vi "Validate-Repair Path.vi"(11 "path in":string) -> (0 "Valid":bool, 1 "Path type":T1=enum."path-abempty", 2 "Segments":string[](array[string]), 3 "path out":string)   [LabVIEW 2013, in "openURI.lvlib" / "URI-Component.Path.lvclass"]
uses:
  URI-Component.Path.lvclass
  path type -- enum.ctl
  utilities/isHEXDigit.vi
  <vilib>/regexp/Match Regular Expression.xnode
  openURI.lvlib
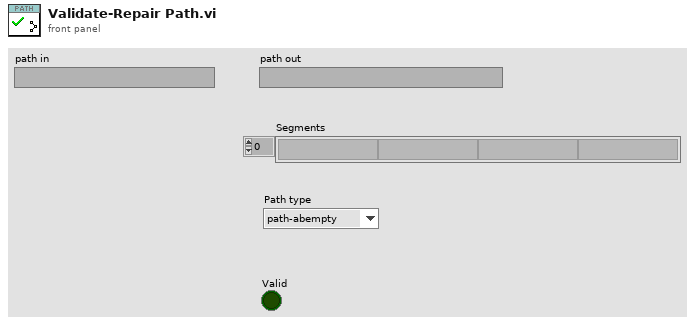
[diagram p1: front panel]
types:
  T1 = typedef "openURI.lvlib/URI-Component.Path.lvclass/path type -- enum.ctl" = enum16{"invalid", "path-abempty", "path-absolute", "path-noscheme", "path-rootless", "path-empty"}
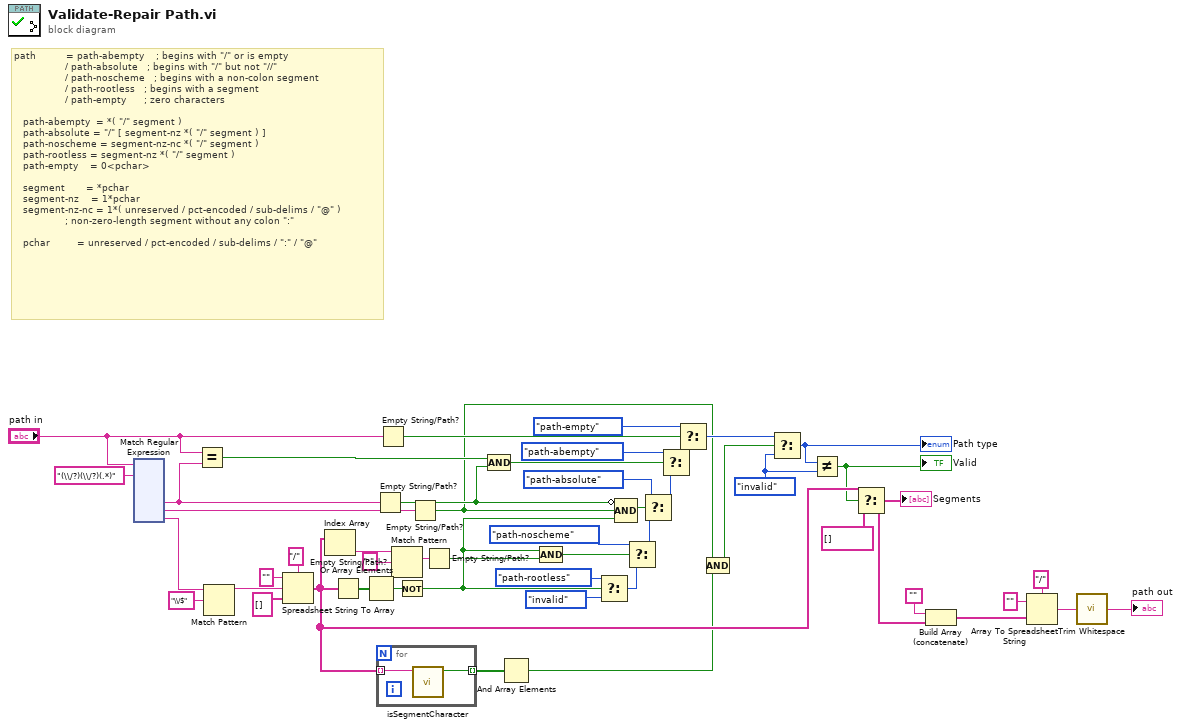
[diagram p0: block diagram]
diagram:
  w49 = path_type_--_enum."invalid" ("path type")
  # "path          = path-abempty    ; begins with \"/\" or is empty\n                 / path-absolute   ; begins with \"/\" but not \"//\"\n                 / path-noscheme   ; begins with a non-colon segment\n                 / path-rootless   ; begins with a segment\n                 / path-empty      ; zero characters\n\n   path-abempty  = *( \"/\" segment )\n   path-absolute = \"/\" [ segment-nz *( \"/\" segment ) ]\n   path-noscheme = segment-nz-nc *( \"/\" segment )\n   path-rootless = segment-nz *( \"/\" segment )\n   path-empty    = 0<pchar>\n\n   segment       = *pchar\n   segment-nz    = 1*pchar\n   segment-nz-nc = 1*( unreserved / pct-encoded / sub-delims / \"@\" )\n                 ; non-zero-length segment without any colon \":\"\n\n   pchar         = unreserved / pct-encoded / sub-delims / \":\" / \"@\""
  n1 = xnode "Match Regular Expression"("input string"="path in", "regular expression"="(\\/?)(\\/?)(.*)") -> ("submatch 1"=w19:string, "submatch 2"=w18:string, "submatch 3"=w40:string)  [unwired: 4 in, 5 out]
  n2 = Equal?(x="path in", y=w19) -> (x = y?=w22:bool)
  n3 = Match Pattern(string=w40, regular expression="\\/$") -> (before substring=w41:string)  [unwired: 1 in, 3 out]
  n4 = Spreadsheet String To Array(delimiter (Tab)="/", format string="", spreadsheet string=w41, array type (2D Dbl)=string[] [] ("Segments")) -> (array=w12:string[])
  n5 = Index Array(array=w12) -> (element=w47:string)  [unwired: 1 in]
  n6 = Empty String/Path?(string/path=w12) -> (empty?=w48:bool[])
  n7 = Or Array Elements(Boolean array=w48) -> (logical OR=w38:bool)
  n8 = Empty String/Path?(string/path=w19) -> (empty?=w34:bool)
  n9 = for {
    tunnel: [w52] -> w15 mode=indexing
    tunnel: w12 -> [w51] mode=indexing
    n10 = call "isSegmentCharacter.vi"("characters"=w51) -> ("pchar"=w52:bool)  [unwired: 10 in]
  }
  n11 = Empty String/Path?(string/path="path in") -> (empty?=w26:bool)
  n12 = Match Pattern(string=w47, regular expression=":" ("string")) -> (match substring=w43:string)  [unwired: 1 in, 3 out]
  n13 = Not(x=w38) -> (.not. x?=w45:bool)
  n14 = Empty String/Path?(string/path=w18) -> (empty?=w14:bool)
  n15 = Empty String/Path?(string/path=w43) -> (empty?=w44:bool)
  n16 = Compound Arithmetic op=AND(w22, w34) -> (w21:bool)
  n17 = And Array Elements(Boolean array=w15) -> (logical AND=w11:bool)
  n18 = Compound Arithmetic op=AND(w45, w44) -> (w46:bool)
  n19 = Select(t=path_type_--_enum."path-rootless" ("path type"), s=w45, f=path_type_--_enum."invalid" ("path type")) -> (s? t:f=w36:T1)
  n20 = Compound Arithmetic op=AND(invert w34, w14, w45) -> (w23:bool)
  n21 = Select(t=path_type_--_enum."path-noscheme" ("path type"), s=w46, f=w36) -> (s? t:f=w33:T1)
  n22 = Select(t=path_type_--_enum."path-absolute" ("path type"), s=w23, f=w33) -> (s? t:f=w25:T1)
  n23 = Select(t=path_type_--_enum."path-abempty" ("path type"), s=w21, f=w25) -> (s? t:f=w50:T1)
  n24 = Select(t=path_type_--_enum."path-empty" ("path type"), s=w26, f=w50) -> (s? t:f=w28:T1)
  n25 = Compound Arithmetic op=AND(w14, w11) -> (w13:bool)
  n26 = Select(t=w28, s=w13, f=w49) -> (s? t:f=w10:T1)
  "Path type" <- w10
  n27 = Not Equal?(x=w10, y=w49) -> (x != y?=w9:bool)
  "Valid" <- w9
  n28 = Select(t=w12, s=w9, f=string[] []) -> (s? t:f=w2:string[])
  "Segments" <- w2
  n29 = Build Array (concatenate)("", w2) -> (w3:string[])
  n30 = Array To Spreadsheet String(delimiter (Tab)="/", array=w3, 3:"" ("format string")) -> (spreadsheet string=w5:string)
  n31 = call <vilib>:"Trim Whitespace.vi"("string"=w5) -> ("trimmed string"=→"path out":string)  [unwired: 1 in]
